vi "数据查询_数据查询.vi"() -> ()   [LabVIEW 2016]
uses:
  <vilib>/Utility/miscctls.llb/LVPointTypeDef.ctl
  <vilib>/Utility/miscctls.llb/LVRowAndColumnUnsignedTypeDef.ctl
  <userlib>/_OpenG.lib/array/array.llb/Sort 2D Array (String)__ogtk.vi
  <vilib>/addons/database/_DB Variant To Data/Database Variant To Data.xnode
panel:
  in  "下拉列表":string(xcontrol)
  in  "导出":bool
  out "分钟小时":string(combo)="实时数据"
  out "工作类型":string(combo)="全部数据"
  out "连接的字符串":string
  out "选中数据表":string
  in  "查询":bool
  in  "结束日期":string="2050/01/01"
  in  "起始日期":string="2010/01/01"
  out "XY图":cluster{"data":timestamp[], "data":dbl[]}[](graph)
  out "数据表":string[][](table)
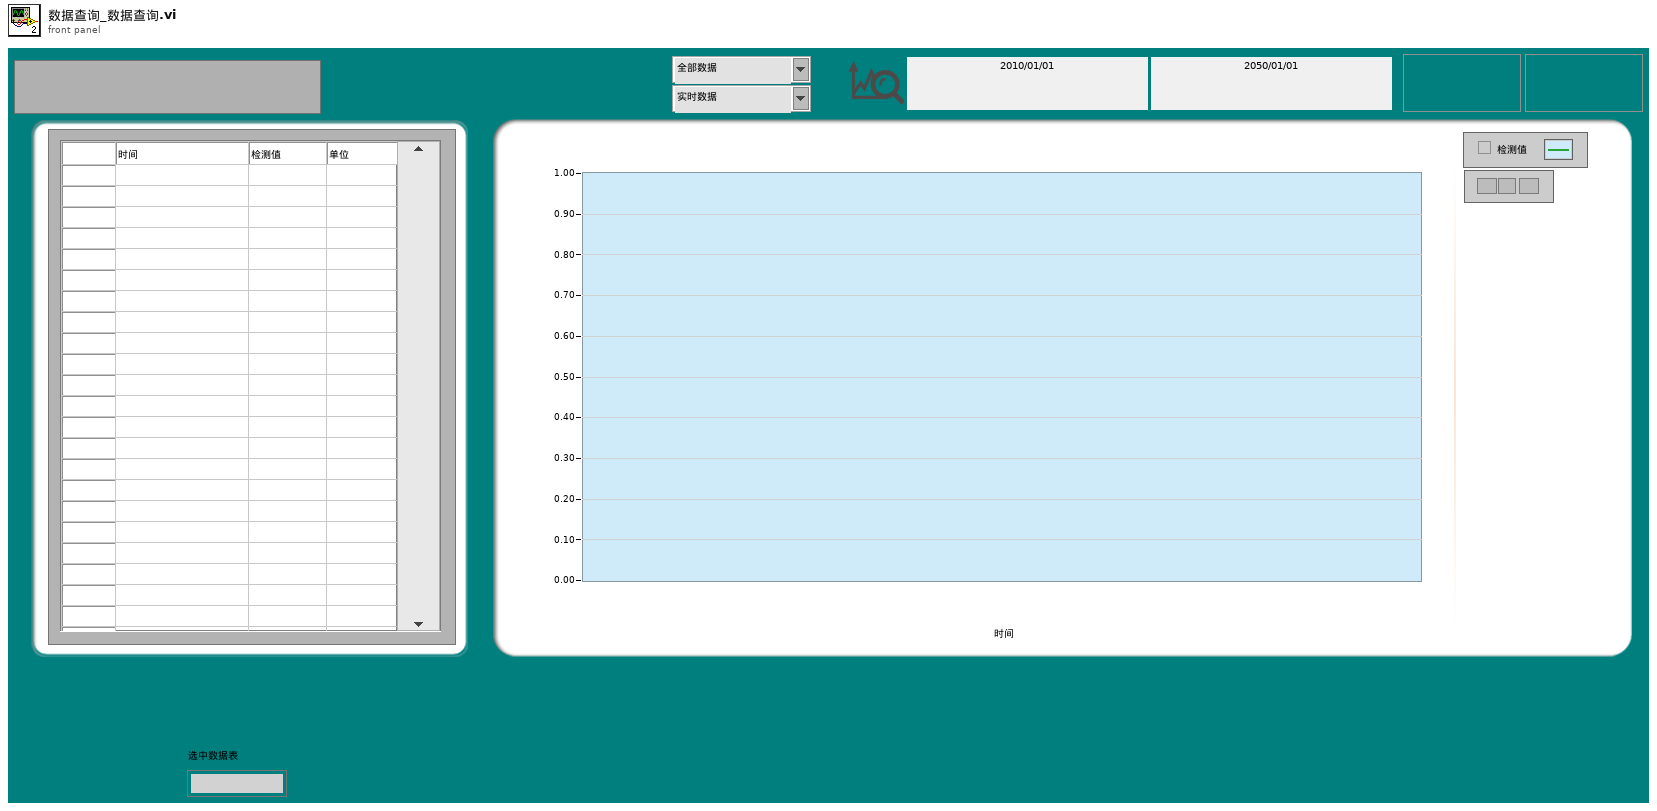
[diagram p1: front panel]
types:
  T1 = typedef "LVPointTypeDef.ctl" = cluster{"Horizontal":i16, "Vertical":i16}
  T2 = typedef "LVDateTimeRec.ctl" = cluster{"秒数的小数部分":dbl, "秒":i32, "分":i32, "时":i32, "日":i32, "月":i32, "年":i32, "天数（周）":i32, "天数（年）":i32, "DST":i32}
  T3 = enum8{"Enabled", "Disabled", "Disabled and Grayed Out"}
  T4 = typedef "LVPoint32TypeDef.ctl" = cluster{"Horizontal":i32, "Vertical":i32}
  T5 = typedef "LVPointDoubleTypeDef.ctl" = cluster{"Cursor X":dbl, "Cursor Y":dbl}
  T6 = typedef "LVRowAndColumnUnsignedTypeDef.ctl" = cluster{"Row":u32, "Column":u32}
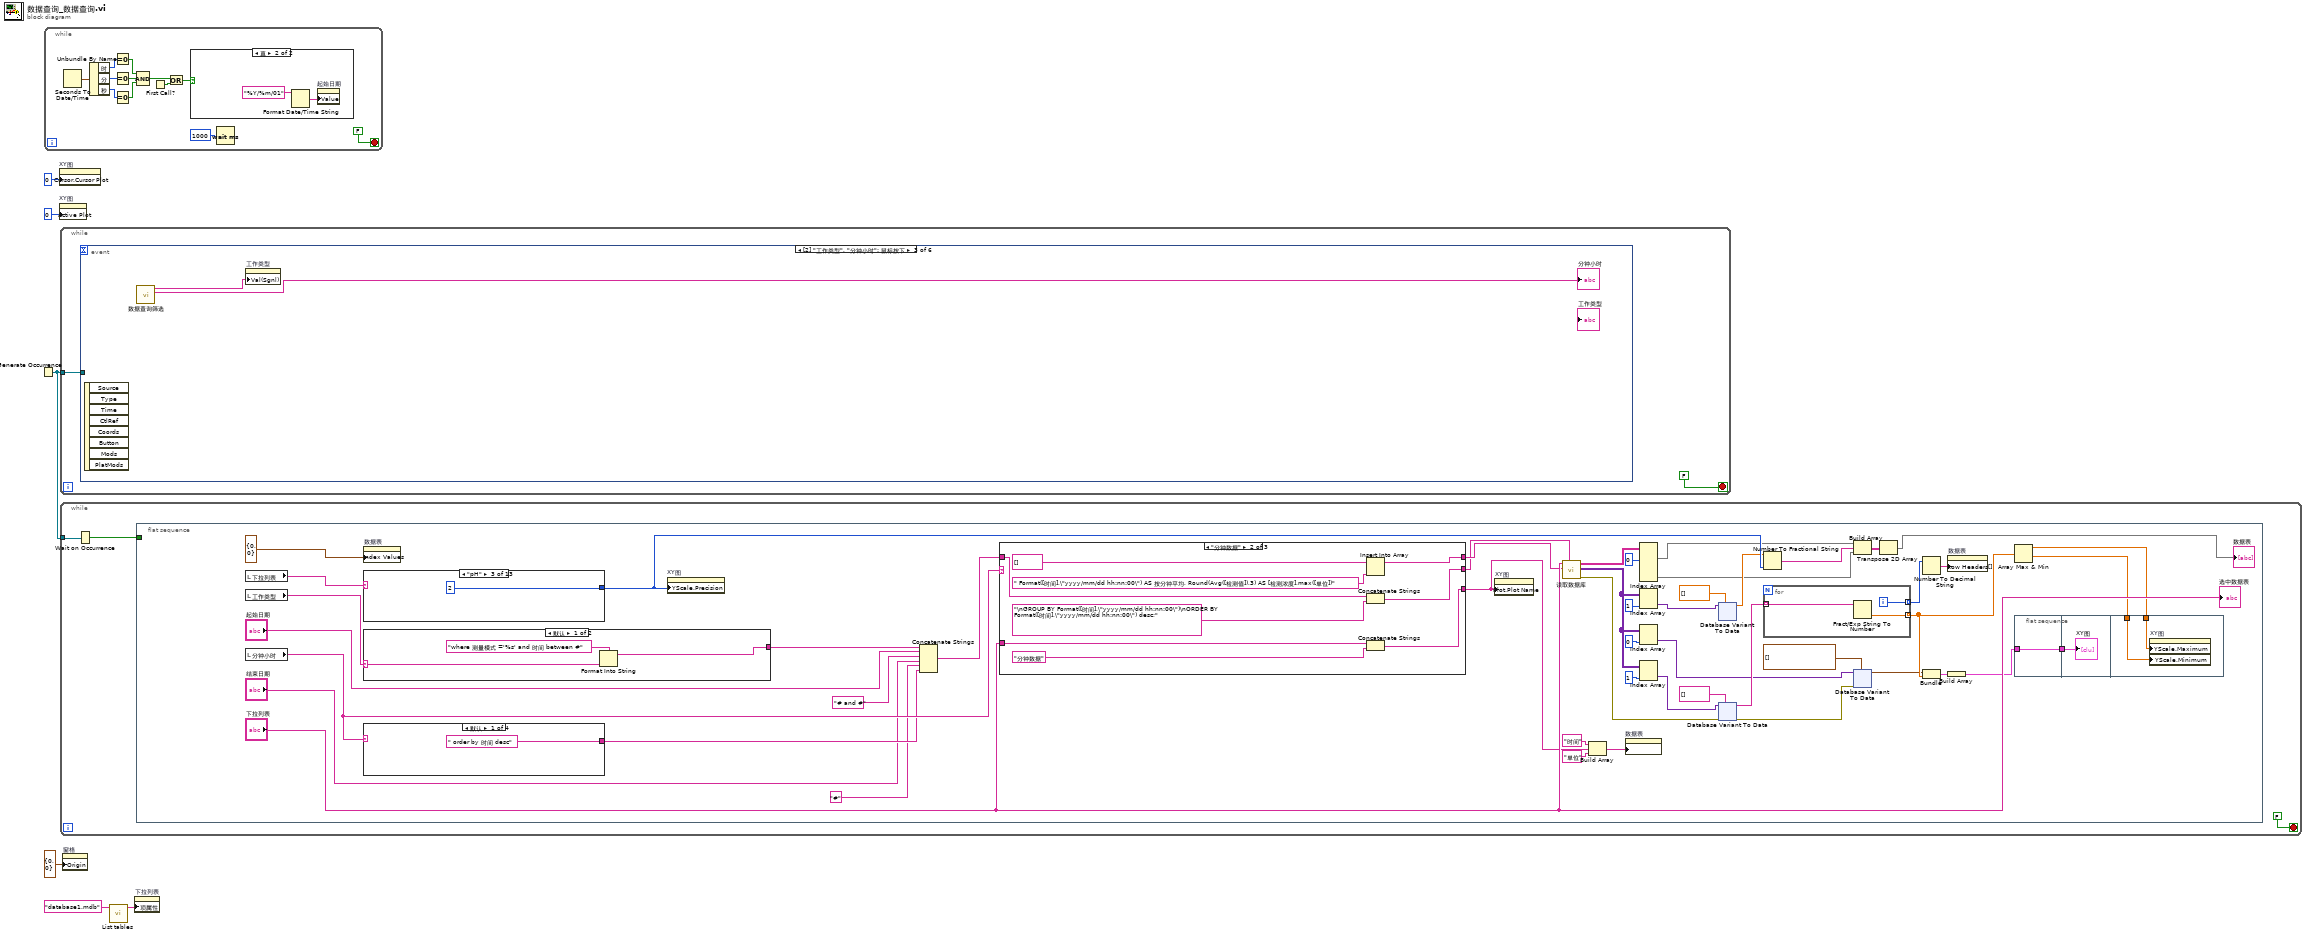
[diagram p0: block diagram]
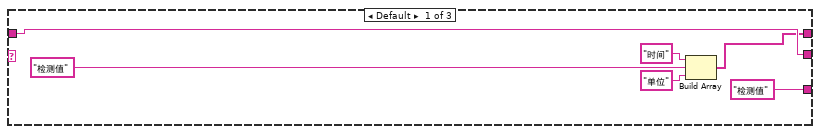
[diagram p2: hidden frame]
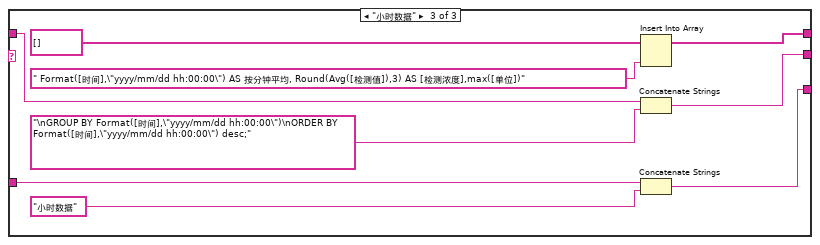
[diagram p3: hidden frame]
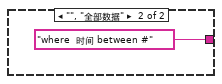
[diagram p7: hidden frame]
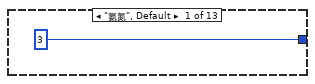
[diagram p8: hidden frame]
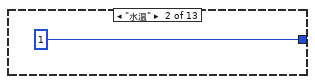
[diagram p9: hidden frame]
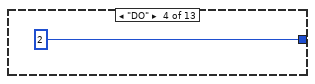
[diagram p10: hidden frame]
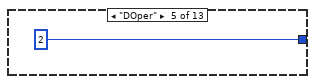
[diagram p11: hidden frame]
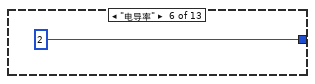
[diagram p12: hidden frame]
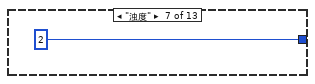
[diagram p13: hidden frame]
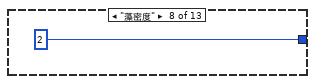
[diagram p14: hidden frame]
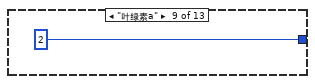
[diagram p15: hidden frame]
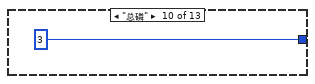
[diagram p16: hidden frame]
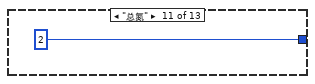
[diagram p17: hidden frame]
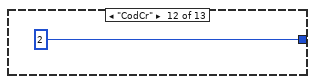
[diagram p18: hidden frame]
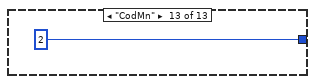
[diagram p19: hidden frame]
diagram:
  n1 = Generate Occurrence() -> (w1:refnum<k4>)
  n2 = while {
    stop <- FALSE stop-if-true
    n3 = Seconds To Date/Time() -> (date time rec=w18:T2)  [unwired: 2 in]
    n4 = Unbundle By Name(w18) -> ("时"=w17:i32, "分"=w16:i32, "秒"=w15:i32)
    n5 = Equal To 0?(x=w17) -> (x = 0?=w14:bool)
    n6 = Equal To 0?(x=w16) -> (x = 0?=w13:bool)
    n7 = Equal To 0?(x=w15) -> (x = 0?=w12:bool)
    n8 = Compound Arithmetic op=AND ("复合运算")(w14, w13, w12) -> (w9:bool)
    n9 = First Call?() -> (First Call?: T/F=w7:bool)
    n10 = Or(x=w9, y=w7) -> (x .or. y?=w8:bool)
    n11 = case shown="真" w8 {
      frame False {
      }
      frame True {
        n12 = Format Date/Time String(time format string (%c)="%Y/%m/01" ("时间格式字符串(%c)")) -> (date/time string=w19:string)  [unwired: 2 in]
        n13 = property on="起始日期" class="Str"("Value"=w19) -> ()  [unwired: 2 in, 2 out]
      }
    }
    n14 = Wait (ms)(milliseconds to wait=u32 1000 ("等待时间（毫秒）")) -> ()  [unwired: 1 out]
  }
  n15 = property on="XY图" class="XYGraph (严格)"("Cursor.Cursor Plot"=0 ("游标.游标关联曲线")) -> ()  [unwired: 2 in, 2 out]
  n16 = property on="XY图" class="XYGraph (严格)"("Active Plot"=u32 0 ("活动曲线")) -> ()  [unwired: 2 in, 2 out]
  n17 = while {
    tunnel: w1 -> [w21]
    stop <- FALSE stop-if-true
    n18 = event shown="[2] \"工作类型\", \"分钟小时\": 鼠标按下" {
      selector: _ -> [_ _ _ _ _ _]
      dyn-events: _ -> [_ _ _ _ _ _]
      timeout: _ -> [_ _ _ _ _ _]
      tunnel: w21 -> [_ _ _ _ w57 _]
      event Timeout {
        n19 = event-data() -> ()  [unwired: 1 in, 3 out]
      }
      event "导出": Value Change {
        n20 = event-data() -> ("CtlRef"=w29:refnum<vi>)  [unwired: 1 in, 5 out]
        n21 = property class="Bool"(reference=w29, "DisabledEnum"=T3."Disabled and Grayed Out" ("禁用")) -> (reference out=w26:refnum<vi>, error out=w27:errorcluster)  [unwired: 1 in]
        n22 = flat-sequence {
          tunnel: w27 -> [_]
          tunnel: [w38] -> w25
          tunnel: w26 -> [w38]
          tunnel: "导出" -> [_]
          frame #0 {
            n23 = local read "数据表"() -> (w46:string[][])
            n24 = property on="数据表" class="Tbl (严格)"() -> ("Column Headers[]"=w31:string[])  [unwired: 2 in, 2 out]
            n25 = call "Removable devices detection v8.5.vi"() -> ("Removable"=w35:string[])  [unwired: 4 out]
            n26 = Insert Into Array(array=string[][] [], new element=w31) -> (w30:string[][])  [unwired: 2 in]
            n27 = Index Array(array=w35) -> (element=w34:string)  [unwired: 1 in]
            n28 = call-poly <userlib>:"Sort Array__ogtk.vi"("Column/Row to Sort By"=u32 0, "Sort By in"=enum16{"row", "column"}."column", "Order"=enum16{"ascending", "descending"}."ascending", "Array in"=w46) -> ("Sorted Array out"=w45:string[][])  [unwired: 4 in, 3 out]
            n29 = String To Path(string=w34) -> (path=w33:path)
            n30 = Index Array(array=w45, index (col)=1 ("禁用的索引 (列)")) -> (element=w41:string[])  [unwired: 1 in]
            n31 = Get Date/Time In Seconds() -> (seconds since 1Jan1904=w48:timestamp)
            n32 = local read "下拉列表"() -> (w39:string)
            n33 = Fract/Exp String To Number(string=w41) -> (number=w40:dbl[])  [unwired: 3 in, 1 out]
            n34 = call "MS Office Report"("Path to Save Report"=w33, "导出日期"=w48, "监测参数"=w39, "数据输入"=w45, "图表输入"=w40, "字段定义"=w30) -> ("error out"=w37:errorcluster)  [unwired: 20 in, 1 out]
            n35 = case shown="错误" w37 {
              tunnel: ["导出成功" ("消息") "导出失败" ("消息")] -> w36
              frame No Error {
              }
              frame Error {
              }
            }
            n36 = One Button Dialog(message=w36) -> ()  [unwired: 1 in, 1 out]
          }
        }
        n37 = property class="Bool"(reference=w25, "DisabledEnum"=T3."Enabled" ("禁用")) -> ()  [unwired: 1 in, 2 out]
      }
      event "工作类型", "分钟小时": Mouse Down {
        n38 = event-data() -> ()  [unwired: 1 in, 8 out]
        n39 = call "数据查询筛选.vi"() -> ("分钟小时"=→"分钟小时":string, "工作类型"=w51:string)  [unwired: 10 in]
        n40 = property on="工作类型" class="CmbBox"("Val(Sgnl)"=w51) -> ()  [unwired: 2 in, 2 out]
      }
      event "起始日期", "结束日期": Mouse Down {
        n41 = event-data() -> ("CtlRef"=w56:refnum<vi>)  [unwired: 1 in, 7 out]
        n42 = property class="Str"(reference=w56) -> (reference out=w54:refnum<vi>, "Value"=w55:string)  [unwired: 1 in, 1 out]
        n43 = call "日期键盘.vi"("原值"=w55) -> ("x+y"=w53:string)  [unwired: 10 in]
        n44 = property class="Str"(reference=w54, "Val(Sgnl)"=w53) -> ()  [unwired: 1 in, 2 out]
      }
      event "查询", "下拉列表", "起始日期", "结束日期", "工作类型", "分钟小时": Value Change {
        n45 = event-data() -> ()  [unwired: 1 in, 6 out]
        n46 = Set Occurrence(w57) -> ()
        n47 = call "List tables.vi"("database"="database1.mdb") -> ("tables"=w58:string[])  [unwired: 9 in, 1 out]
        n48 = property on="下拉列表" class="下拉列表 (严格)"("项属性"=w58) -> ()  [unwired: 2 in, 2 out]
      }
      event "XY图": Mouse Move {
        w64 = "   " ("字符串")
        n49 = event-data() -> ("CtlRef"=w74:refnum<vi>, "Coords"=w73:T4)  [unwired: 1 in, 3 out]
        n50 = invoke class="XYGraph (严格)" method="Map Coords To XY"(reference=w74, "Coords"=w73) -> (reference out=w72:refnum<vi>, error out=w69:errorcluster, "XY"=w71:cluster{"X":dbl, "Y":dbl})  [unwired: 5 in, 4 out]
        n51 = property class="XYGraph (严格)"(reference=w72, error in=w69, "Cursor.Cursor Position"=w71) -> (error out=w70:errorcluster)  [unwired: 1 out]
        n52 = property on="XY图" class="XYGraph (严格)"(error in=w70) -> ("Cursor.Cursor Position"=w67:T5, "YScale.Precision"=w60:u8)  [unwired: 1 in, 2 out]
        n53 = Unbundle(w67) -> ("Cursor X"=w66:dbl, "Cursor Y"=w63:dbl)
        n54 = Format Date/Time String(seconds (now)=w66) -> (date/time string=w65:string)  [unwired: 2 in]
        n55 = Number To Fractional String(number=w63, precision (6)=w60) -> (F-format string=w62:string)  [unwired: 2 in]
        n56 = property on="XY图" class="XYGraph (严格)"() -> ("Plot.Plot Name"=w61:string)  [unwired: 2 in, 2 out]
        n57 = Concatenate Strings(w61, w64, w65, w64, w62) -> (→"连接的字符串":string)
      }
    }
  }
  n58 = while {
    tunnel: w1 -> [w76]
    stop <- FALSE stop-if-true
    n59 = Wait on Occurrence(2:w76) -> (0:w75:bool)  [unwired: 2 in]
    n60 = flat-sequence {
      tunnel: w75 -> [_]
      frame #0 {
        n61 = local read "下拉列表"() -> (w110:string)
        n62 = local read "工作类型"() -> (w115:string)
        n63 = local read "分钟小时"() -> (w119:string)
        n64 = property on="数据表" class="Tbl (严格)"("Index Values"=T6 {"Row"=0, "Column"=0} ("索引值")) -> ()  [unwired: 2 in, 2 out]
        n65 = case shown="\"pH\"" w110 {
          tunnel: [i16 3 ("精度(6)") i16 1 ("精度(6)") i16 2 ("精度(6)") i16 2 ("精度(6)") i16 2 ("精度(6)") i16 2 ("精度(6)") i16 2 ("精度(6)") i16 2 ("精度(6)") i16 2 ("精度(6)") i16 3 ("精度(6)") i16 2 ("精度(6)") i16 2 ("精度(6)") i16 2 ("精度(6)")] -> w114
          frame "氨氮", Default {
          }
          frame "水温" {
          }
          frame "pH" {
          }
          frame "DO" {
          }
          frame "DOper" {
          }
          frame "电导率" {
          }
          frame "浊度" {
          }
          frame "藻密度" {
          }
          frame "叶绿素a" {
          }
          frame "总磷" {
          }
          frame "总氮" {
          }
          frame "CodCr" {
          }
          frame "CodMn" {
          }
        }
        n66 = case shown="默认" w115 {
          selector: w115 -> [w154 _]
          tunnel: [w152 "where  时间 between #" ("condition")] -> w116
          frame Default {
            n67 = Format Into String(format string="where 测量模式 ='%s' and 时间 between #" ("condition"), w154) -> (resulting string=w152:string)  [unwired: 2 in, 1 out]
          }
          frame "", "全部数据" {
          }
        }
        n68 = case shown="默认" w119 {
          tunnel: [" order by 时间 desc" ("字符串") _ _ _] -> w117
          frame Default {
          }
          frame "分钟数据" {
          }
          frame "小时数据" {
          }
          frame "真" {
          }
        }
        n69 = property on="XY图" class="XYGraph (严格)"("YScale.Precision"=w114) -> ()  [unwired: 2 in, 2 out]
        n70 = Concatenate Strings(w116, "起始日期", "# and #" ("condition"), "结束日期", "#" ("condition"), w117) -> (w118:string)
        n71 = case shown="\"分钟数据\"" w119 {
          tunnel: [w128 w140 w145] -> w121
          tunnel: w118 -> [w132 w138 w147]
          tunnel: [w132 w137 w146] -> w120
          tunnel: ["检测值" w133 w142] -> w122
          tunnel: "下拉列表" -> [_ w134 w144]
          frame Default {
            n72 = Build Array("时间", "检测值", "单位" ("元素")) -> (w128:string[])
          }
          frame "分钟数据" {
            n73 = Insert Into Array(array=string[] [] ("显示项"), new element=" Format([时间],\"yyyy/mm/dd hh:nn:00\") AS 按分钟平均, Round(Avg([检测值]),3) AS [检测浓度],max([单位])" ("新元素/子数组")) -> (w140:string[])  [unwired: 1 in]
            n74 = Concatenate Strings(w138, "\nGROUP BY Format([时间],\"yyyy/mm/dd hh:nn:00\")\nORDER BY Format([时间],\"yyyy/mm/dd hh:nn:00\") desc;" ("字符串")) -> (w137:string)
            n75 = Concatenate Strings(w134, "分钟数据" ("字符串")) -> (w133:string)
          }
          frame "小时数据" {
            n76 = Insert Into Array(array=string[] [] ("显示项"), new element=" Format([时间],\"yyyy/mm/dd hh:00:00\") AS 按分钟平均, Round(Avg([检测值]),3) AS [检测浓度],max([单位])" ("新元素/子数组")) -> (w145:string[])  [unwired: 1 in]
            n77 = Concatenate Strings(w147, "\nGROUP BY Format([时间],\"yyyy/mm/dd hh:00:00\")\nORDER BY Format([时间],\"yyyy/mm/dd hh:00:00\") desc;" ("字符串")) -> (w146:string)
            n78 = Concatenate Strings(w144, "小时数据" ("字符串")) -> (w142:string)
          }
        }
        n79 = property on="XY图" class="XYGraph (严格)"("Plot.Plot Name"=w122) -> ()  [unwired: 2 in, 2 out]
        n80 = call "读取数据库.vi"("condition"=w120, "显示项"=w121, "组合框"="下拉列表") -> ("error out"=w87:errorcluster, "data"=w103:variant[][], "表格"=w93:string[][])  [unwired: 5 in, 1 out]
        n81 = Build Array("时间", w122, "单位" ("元素")) -> (w99:string[])
        n82 = property on="数据表" class="Tbl (严格)"("Column Headers[]"=w99) -> ()  [unwired: 2 in, 2 out]
        n83 = Index Array(array=w93, index (col) #1=0 ("禁用的索引 (列)")) -> (element #1=w95:string[], element #3=w102:string[])  [unwired: 5 in, 1 out]
        n84 = Index Array(array=w103, index (col)=1 ("禁用的索引 (列)")) -> (element=w105:variant[])  [unwired: 1 in]
        n85 = Index Array(array=w103, index (col)=0 ("禁用的索引 (列)")) -> (element=w84:variant[])  [unwired: 1 in]
        n86 = Index Array(array=w103, index (col)=1 ("禁用的索引 (列)")) -> (element=w86:variant[])  [unwired: 1 in]
        n87 = xnode "Database Variant To Data"("database variant"=w105, "type"=sgl[] []) -> ("data"=w107:sgl[])  [unwired: 1 in, 1 out]
        n88 = xnode "Database Variant To Data"("database variant"=w86, "error in (no error)"=w87, "type"=string[] []) -> ("data"=w100:string[], "error out"=w88:errorcluster)
        n89 = Number To Fractional String(number=w107, precision (6)=w114) -> (F-format string=w108:string[])  [unwired: 2 in]
        n90 = for {
          tunnel: w100 -> [w209] mode=indexing
          tunnel: [w208] -> w111 mode=indexing
          tunnel: [w207] -> w123 mode=indexing
          i -> [w207]
          n91 = Fract/Exp String To Number(string=w209) -> (number=w208:dbl)  [unwired: 3 in, 1 out]
        }
        n92 = Build Array(w95, w108, w102) -> (w96:string[][])
        n93 = xnode "Database Variant To Data"("database variant"=w84, "error in (no error)"=w88, "type"=timestamp[] []) -> ("data"=w92:timestamp[])  [unwired: 1 out]
        n94 = Transpose 2D Array(2D array=w96) -> (transposed array=→"数据表":string[][])
        n95 = Number To Decimal String(number=w123) -> (decimal integer string=w124:string[])  [unwired: 1 in]
        n96 = Bundle("data"=w92, w111) -> (w91:cluster{"data":timestamp[], dbl[]})  [unwired: 1 in]
        n97 = property on="数据表" class="Tbl (严格)"("Row Headers[]"=w124) -> ()  [unwired: 2 in, 2 out]
        n98 = Build Array(w91) -> (w90:cluster{"data":timestamp[], dbl[]}[])
        n99 = Array Max & Min(array=w111) -> (max value=w112:dbl, min value=w113:dbl)  [unwired: 2 out]
        n100 = flat-sequence {
          tunnel: [w210] -> w126
          tunnel: w90 -> [w210]
          tunnel: w126 -> [w211]
          tunnel: w112 -> [w213]
          tunnel: w113 -> [w212]
          frame #0 {
          }
          frame #1 {
            "XY图" <- w211
          }
          frame #2 {
            n101 = property on="XY图" class="XYGraph (严格)"("YScale.Maximum"=w213, "YScale.Minimum"=w212) -> ()  [unwired: 2 in, 2 out]
          }
        }
        "选中数据表" <- "下拉列表"
      }
    }
  }
  n102 = property on="窗格" class="Pane"("Origin"=T1 {"Horizontal"=0, "Vertical"=0} ("原点")) -> ()  [unwired: 2 in, 2 out]
  n103 = call "List tables.vi"("database"="database1.mdb") -> ("tables"=w2:string[])  [unwired: 9 in, 1 out]
  n104 = property on="下拉列表" class="下拉列表 (严格)"("项属性"=w2) -> ()  [unwired: 2 in, 2 out]
